vi "RT_Thrust_Force_in_DLR_Navigation_Reference_System(SubVI).vi"(9 "DCM":dbl[][](array[numeric]), 10 "FE_b":dbl[](array[numeric])) -> (3 "FE":dbl[](array[numeric]))   [LabVIEW 2017]
uses:
  <vilib>/Analysis/baseanly.llb/Real A x B.vi
  <vilib>/Analysis/Matrix/Numeric/Conversions/Array To Matrix - RA.vi
  <vilib>/Analysis/Matrix/Numeric/Conversions/Array To Matrix - RA2.vi
  <vilib>/Analysis/Matrix/Numeric/Conversions/Matrix To Array - RM.vi
  <vilib>/Analysis/Matrix/NI_Matrix.lvlib
  <vilib>/Analysis/NI_AALBase.lvlib
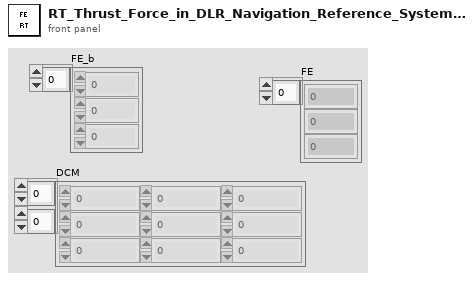
[diagram p1: front panel]
types:
  T1 = typedef "NI_Matrix.lvlib/RealMatrix.ctl" = dbl[][]
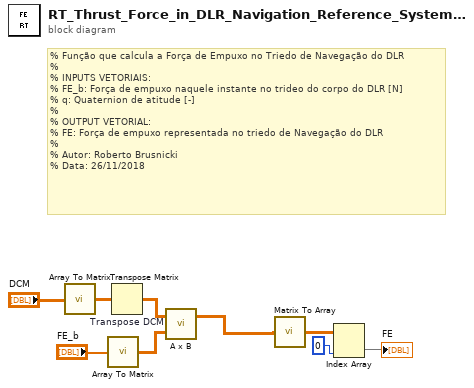
[diagram p0: block diagram]
diagram:
  # "% Função que calcula a Força de Empuxo no Triedo de Navegação do DLR \n%\n% INPUTS VETORIAIS:\n% FE_b: Força de empuxo naquele instante no trideo do corpo do DLR [N]\n% q: Quaternion de atitude\t[-]\n%\n% OUTPUT VETORIAL:\n% FE: Força de empuxo representada no triedo de Navegação do DLR\n%\n% Autor: Roberto Brusnicki\n% Data: 26/11/2018"
  n1 = call-poly <vilib>:"Array To Matrix.vi"("Real 2D Array"="DCM") -> ("Real Matrix"=w4:T1)
  n2 = call-poly <vilib>:"Array To Matrix.vi"("Real 1D Array"="FE_b") -> ("Real Matrix (Column Vector)"=w6:T1)
  n3 = Transpose Matrix "Transpose DCM"(1:w4) -> (0:w5:T1)
  n4 = call-poly <vilib>:"A x B.vi"("B"=w6, "A"=w5) -> ("A x B"=w3:T1)  [unwired: 1 out]
  n5 = call-poly <vilib>:"Matrix To Array.vi"("Real Matrix"=w3) -> ("Real 2D Array"=w9:dbl[][])
  n6 = Index Array(array=w9, index (col)=0 ("index (row)")) -> (element=→"FE":dbl[])  [unwired: 1 in]
